vi "ReadTextFiles2ExcelCSV_Subvi.vi"(8 "error out":errorcluster, 9 "Array":string[](array[string]), 10 "Run Number":string, 11 "base path":path=path "D:/SEE_Campaigns/TAMU_AUG_2024/Outputs/SundayTAMU2024") -> (0 "error out 2":errorcluster)   [LabVIEW 2019]
uses:
  <vilib>/Utility/file.llb/Write Delimited Spreadsheet (string).vi
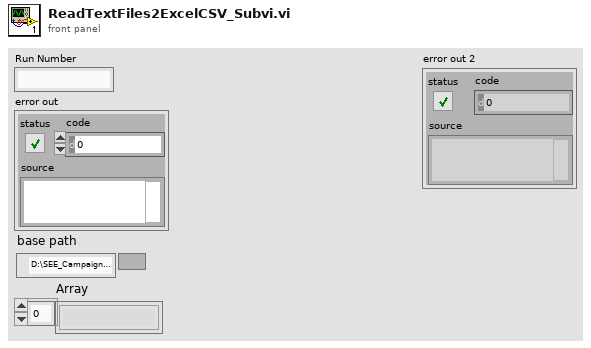
[diagram p1: front panel]
types:
  T1 = enum16{"open", "replace", "create", "open or create", "replace or create", "replace or create with confirmation"}
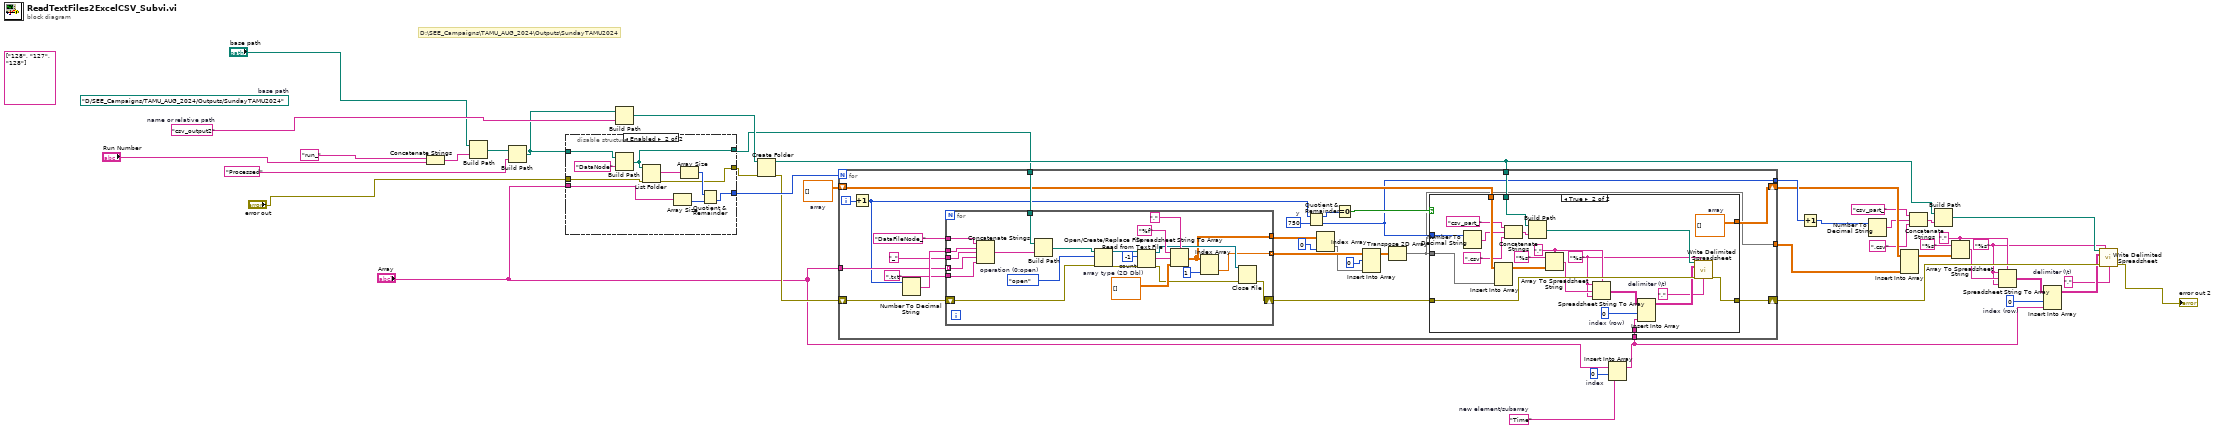
[diagram p0: block diagram]
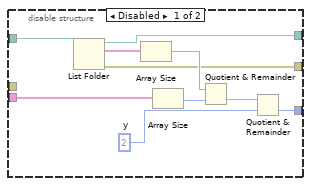
[diagram p2: hidden frame]
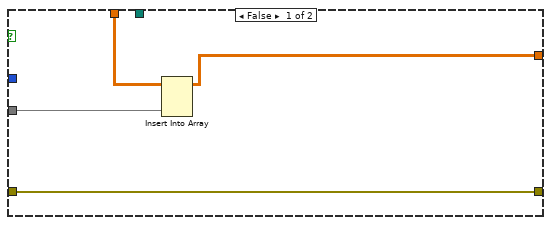
[diagram p3: hidden frame]
diagram:
  w6 = "Time"  # new element/subarray
  w7 = 0  # index
  w8 = ","  # delimiter (\t)
  w9 = 0  # index (row)
  w12 = "%s" ("format (%.3f)")
  w14 = "," ("delimiter (Tab)")
  w30 = dbl[][] []  # array
  (unwired) string[] ["128", "127", "128"]
  w39 = "csv_output2"  # name or relative path
  (unwired) path "D:/SEE_Campaigns/TAMU_AUG_2024/Outputs/SundayTAMU2024"  # base path
  # "D:\\SEE_Campaigns\\TAMU_AUG_2024\\Outputs\\SundayTAMU2024"
  n1 = Concatenate Strings("run_" ("string"), "Run Number") -> (w35:string)
  n2 = Build Path(base path="base path", name or relative path=w35) -> (appended path=w34:path)
  n3 = Build Path(base path=w34, name or relative path="Processed") -> (appended path=w4:path)
  n4 = disable-structure shown="Enabled" {
    disable-tunnel: w4 -> [w47 w60]
    disable-tunnel: [w44 w54] -> w33
    disable-tunnel: [w43 w55] -> w32
    disable-tunnel: "Array" -> [w42 w56]
    disable-tunnel: [w41 w52] -> w3
    disable-tunnel: "error out" -> [_ w51]
    frame Disabled {
      w45 = 2  # y
      n5 = List Folder(path=w47) -> (path out=w41:path, filenames=w50:string[], error out=w43:errorcluster)  [unwired: 3 in, 1 out]
      n6 = Array Size(array=w50) -> (size(s)=w48:i32)
      n7 = Array Size(array=w42) -> (size(s)=w49:i32)
      n8 = Quotient & Remainder(x=w48, y=w49) -> (floor(x/y)=w46:i32)  [unwired: 1 out]
      n9 = Quotient & Remainder(x=w46, y=w45) -> (floor(x/y)=w44:i32)  [unwired: 1 out]
    }
    frame Enabled {
      n10 = Build Path(base path=w60, name or relative path="DataNode") -> (appended path=w52:path)
      n11 = List Folder(path=w52, error in=w51) -> (filenames=w59:string[], error out=w55:errorcluster)  [unwired: 2 in, 2 out]
      n12 = Array Size(array=w56) -> (size(s)=w58:i32)
      n13 = Array Size(array=w59) -> (size(s)=w57:i32)
      n14 = Quotient & Remainder(x=w57, y=w58) -> (floor(x/y)=w54:i32)  [unwired: 1 out]
    }
  }
  n15 = Build Path(base path=w4, name or relative path=w39) -> (appended path=w29:path)
  n16 = Create Folder(path (use dialog)=w29, error in=w32) -> (created path=w23:path, error out=w31:errorcluster)  [unwired: 1 in, 1 out]
  n17 = Insert Into Array(array="Array", index=w7, new element=w6) -> (w5:string[])
  n18 = for {
    N: w33 -> [_]
    tunnel: "Array" -> [w83]
    shift-right: [w67] -> w26
    shift-left: w31 -> [w80]
    tunnel: w3 -> [w81]
    shift-right: [w66] -> w25
    shift-left: w30 -> [w69]
    tunnel: w23 -> [w65]
    tunnel: w5 -> [w63]
    tunnel: [w62] -> w28
    tunnel: [w61] -> w24
    i -> [w74]
    w72 = 750  # y
    n19 = Increment(x=w74) -> (x+1=w73:i32)
    n20 = Number To Decimal String(number=w73) -> (decimal integer string=w86:string)  [unwired: 1 in]
    n21 = for {
      tunnel: w83 -> [w132] mode=indexing
      tunnel: w86 -> [w135]
      tunnel: "DataFileNode_" -> [w134]
      tunnel: "_" -> [w133]
      tunnel: ".txt" ("string") -> [w131]
      tunnel: w81 -> [w129]
      shift-right: [w115] -> w68
      shift-left: w80 -> [w126]
      tunnel: [w114] -> w77 mode=indexing
      tunnel: [w113] -> w79
      w120 = dbl[][] []  # array type (2D Dbl)
      w123 = -1  # count
      w127 = T1."open"  # operation (0:open)
      n22 = Concatenate Strings(w134, w135, w133, w132, w131) -> (w130:string)
      n23 = Build Path(base path=w129, name or relative path=w130) -> (appended path=w128:path)
      n24 = Open/Create/Replace File(file path (use dialog)=w128, error in=w126, operation (0:open)=w127) -> (refnum out=w125:refnum<file>, error out=w124:errorcluster)  [unwired: 3 in, 1 out]
      n25 = Read from Text File(file (use dialog)=w125, count=w123, error in=w124) -> (refnum out=w117:refnum<file>, text=w122:string, error out=w116:errorcluster)  [unwired: 1 in, 1 out]
      n26 = Spreadsheet String To Array(delimiter (Tab)=",", format string="%f", spreadsheet string=w122, array type (2D Dbl)=w120) -> (array=w113:dbl[][])
      n27 = Index Array(array=w113, index (col)=1 ("disabled index (col)")) -> (element=w114:dbl[])  [unwired: 1 in]
      n28 = Close File(refnum=w117, error in=w116) -> (error out=w115:errorcluster)  [unwired: 1 out]
    }
    n29 = Quotient & Remainder(x=w73, y=w72) -> (x-y*floor(x/y)=w71:i32, floor(x/y)=w62:i32)
    n30 = Index Array(array=w79, index (col)=0 ("disabled index (col)")) -> (element=w76:dbl[])  [unwired: 1 in]
    n31 = Equal To 0?(x=w71) -> (x = 0?=w70:bool)
    n32 = Insert Into Array(array=w77, index (row)=0 ("disabled index (col)"), new element=w76) -> (w75:dbl[][])  [unwired: 1 in]
    n33 = Transpose 2D Array(2D array=w75) -> (transposed array=w61:dbl[][])
    n34 = case shown="True" w70 {
      tunnel: w61 -> [w89 w112]
      tunnel: w69 -> [w90 w111]
      tunnel: w62 -> [_ w107]
      tunnel: w68 -> [w88 w104]
      tunnel: [w88 w103] -> w67
      tunnel: [w87 w102] -> w66
      tunnel: w65 -> [_ w101]
      tunnel: w63 -> [_ w94]
      frame False {
        n35 = Insert Into Array(array=w90, new element=w89) -> (w87:dbl[][])  [unwired: 2 in]
      }
      frame True {
        w91 = ","  # delimiter (\t)
        w92 = 0  # index (row)
        w96 = "%s" ("format (%.3f)")
        w98 = "," ("delimiter (Tab)")
        w102 = dbl[][] []  # array
        n36 = Number To Decimal String(number=w107) -> (decimal integer string=w109:string)  [unwired: 1 in]
        n37 = Insert Into Array(array=w111, new element=w112) -> (w100:dbl[][])  [unwired: 2 in]
        n38 = Concatenate Strings("csv_part_", w109, ".csv") -> (w106:string)
        n39 = Build Path(base path=w101, name or relative path=w106) -> (appended path=w105:path)
        n40 = Array To Spreadsheet String(delimiter (Tab)=w98, array=w100, 3:"%s" ("format string")) -> (spreadsheet string=w97:string)
        n41 = Spreadsheet String To Array(delimiter (Tab)=w98, format string=w96, spreadsheet string=w97, array type (2D Dbl)=w96) -> (array=w95:string[][])
        n42 = Insert Into Array(array=w95, index (row)=w92, new element=w94) -> (w93:string[][])  [unwired: 1 in]
        n43 = call-poly <vilib>:"Write Delimited Spreadsheet.vi"("file path (dialog if empty)"=w105, "format (%s)"=w96, "2D data"=w93, "error in (no error)"=w104, "delimiter (\\t)"=w91) -> ("error out"=w103:errorcluster)  [unwired: 9 in, 1 out]
      }
    }
  }
  n44 = Increment(x=w28) -> (x+1=w27:i32)
  n45 = Number To Decimal String(number=w27) -> (decimal integer string=w20:string)  [unwired: 1 in]
  n46 = Insert Into Array(array=w25, new element=w24) -> (w16:dbl[][])  [unwired: 2 in]
  n47 = Concatenate Strings("csv_part_", w20, ".csv") -> (w18:string)
  n48 = Build Path(base path=w23, name or relative path=w18) -> (appended path=w17:path)
  n49 = Array To Spreadsheet String(delimiter (Tab)=w14, array=w16, 3:"%s" ("format string")) -> (spreadsheet string=w13:string)
  n50 = Spreadsheet String To Array(delimiter (Tab)=w14, format string=w12, spreadsheet string=w13, array type (2D Dbl)=w12) -> (array=w11:string[][])
  n51 = Insert Into Array(array=w11, index (row)=w9, new element=w5) -> (w10:string[][])  [unwired: 1 in]
  n52 = call-poly <vilib>:"Write Delimited Spreadsheet.vi"("file path (dialog if empty)"=w17, "format (%s)"=w12, "2D data"=w10, "error in (no error)"=w26, "delimiter (\\t)"=w8) -> ("error out"=→"error out 2":errorcluster)  [unwired: 9 in, 1 out]
